vi "Send Autosampler Move Needle.vi"(7 "Message Priority (Normal)":T2=enum."Normal", 8 "error in (no error)":errorcluster, 9 "Correlation ID":u32, 10 "Needle Position":T1, 11 "Message Enqueuer":refnum<class "Message Enqueuer.lvclass">) -> (0 "error out":errorcluster, 3 "Message Enqueuer out":refnum<class "Message Enqueuer.lvclass">)   [LabVIEW 2023, in "Application.lvlib" / "Autosampler Move Needle Msg.lvclass"]
doc: "This VI sends the message to an actor."
uses:
  Autosampler Move Needle Msg.lvclass
  <vilib>/ActorFramework/Message Enqueuer/Message Enqueuer.lvclass
  <vilib>/ActorFramework/Message Enqueuer/Message Priority.ctl
  Hardware/Autosampler/Autosampler Needle Position.ctl
  C:/Program Files/National Instruments/LabVIEW 2023/vi.lib/ActorFramework/Message/Message.lvclass
  Autosampler Move Needle Msg.lvclass/Autosampler Move Needle Msg.ctl
  <vilib>/ActorFramework/Message Enqueuer/Message Enqueuer.lvclass/Message Enqueuer.ctl
  <vilib>/ActorFramework/Message Priority Queue/Priority Enqueue.vi
  Hardware/Autosampler/Autosampler.lvlib
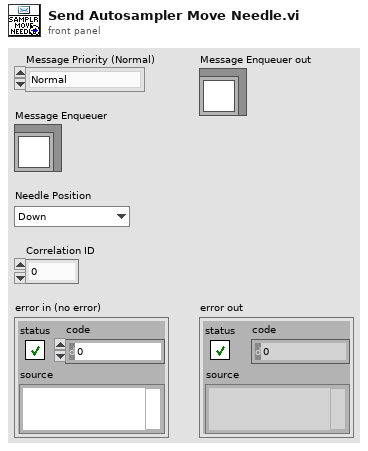
[diagram p1: front panel]
types:
  T1 = typedef "Autosampler.lvlib/Autosampler Needle Position.ctl" = enum16{"Down", "Up"}
  T2 = typedef "Actor Framework.lvlib/Message Enqueuer.lvclass/Message Priority.ctl" = enum16{"Low", "Normal", "High"}
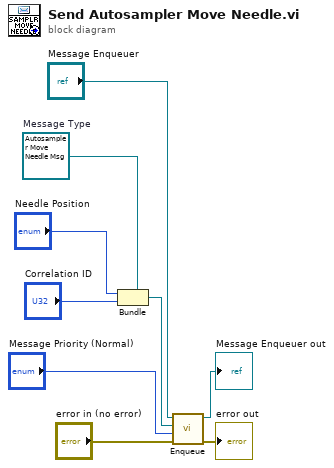
[diagram p0: block diagram]
diagram:
  w3 = refnum<class "Autosampler Move Needle Msg.lvclass"> refnum  # Message Type
  n1 = Bundle(cluster=w3, "Needle Position", "Correlation ID") -> (w4:refnum<class "Autosampler Move Needle Msg.lvclass">)
  n2 = call <vilib>:"Enqueue.vi"("error in (no error)"="error in (no error)", "Message Priority (Normal)"="Message Priority (Normal)", "Message"=w4, "Message Enqueuer in"="Message Enqueuer") -> ("error out"=→"error out":errorcluster, "Message Enqueuer out"=→"Message Enqueuer out":refnum<class "Message Enqueuer.lvclass">)  [unwired: 6 in]
